vi "duty cycle.vi"(4 "State":i16, 5 "Time":dbl format="%.2f", 6 "Sensor Values":dbl[](array[numeric]), 7 "Set Points":dbl[](array[numeric])) -> (0 "required data":T1={"Set Point names"=["on time (s)", "off time (s)", "on value"], "required number of setpoints"=3, "required number of sensors"=1, "Sensor names"=["elapsed time"]}, 3 "output value":dbl)   [LabVIEW 2010]
panel:
  # "Enter the correct information for this control code in the required data structure below. Then make the current value default by right clicking on the border of the data structure. Select \"data operations\" and then select \"make current value default\". These values will be displayed by process controller."
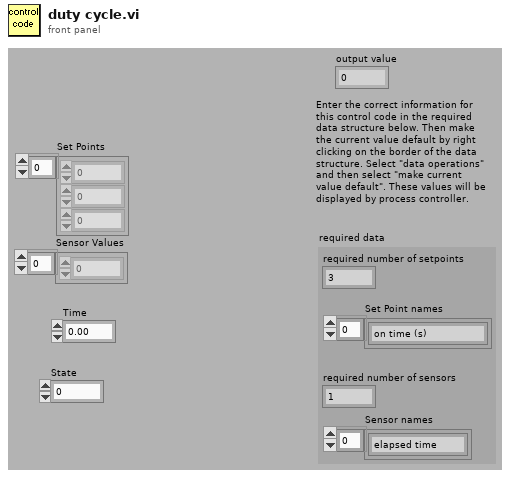
[diagram p1: front panel]
types:
  T1 = cluster{"Set Point names":string[], "required number of setpoints":u8, "required number of sensors":u8, "Sensor names":string[]}
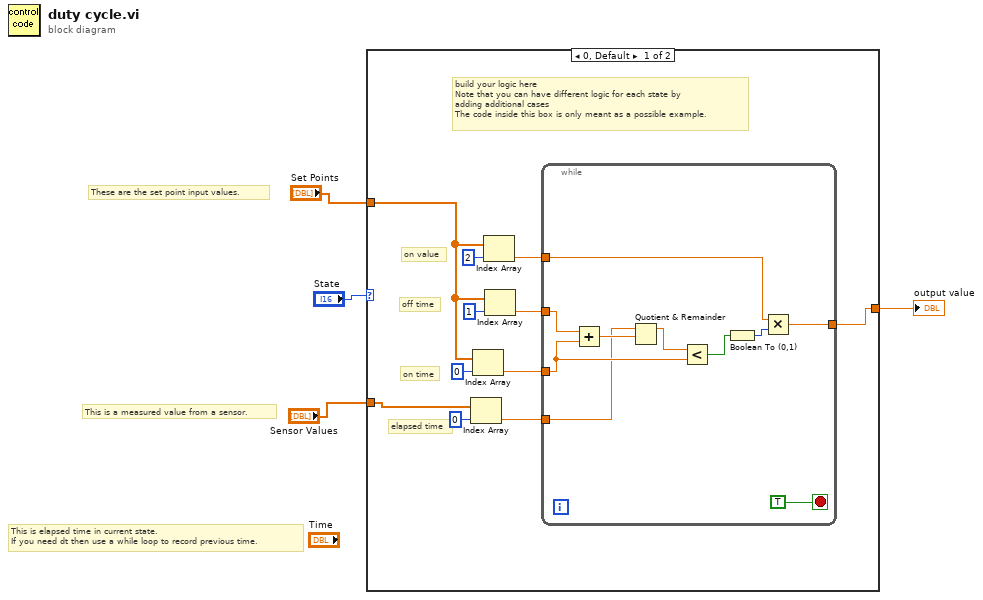
[diagram p0: block diagram]
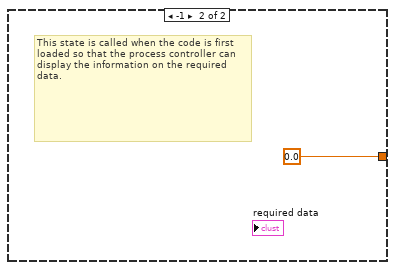
[diagram p2: hidden frame]
diagram:
  # "These are the set point input values."
  # "This is a measured value from a sensor."
  # "This is elapsed time in current state.\nIf you need dt then use a while loop to record previous time."
  n1 = case shown="0, Default" "State" {
    tunnel: [w8 0.0 ("fraction on")] -> w3
    tunnel: "Set Points" -> [w10 _]
    tunnel: "Sensor Values" -> [w6 _]
    frame 0, Default {
      # "elapsed time"
      # "on value"
      # "off time"
      # "on time"
      # "build your logic here\nNote that you can have different logic for each state by\nadding additional cases\nThe code inside this box is only meant as a possible example."
      n2 = Index Array(array=w6, index=0) -> (element=w5:dbl)
      n3 = Index Array(array=w10, index=0) -> (element=w12:dbl)
      n4 = Index Array(array=w10, index=2) -> (element=w9:dbl)
      n5 = Index Array(array=w10, index=1) -> (element=w14:dbl)
      n6 = while {
        tunnel: w14 -> [w24]
        tunnel: w12 -> [w22]
        tunnel: w9 -> [w19]
        tunnel: [w18] -> w8
        tunnel: w5 -> [w16]
        stop <- TRUE stop-if-true
        n7 = Add(x=w24, y=w22) -> (x+y=w23:dbl)
        n8 = Quotient & Remainder(x=w16, y=w23) -> (x-y*floor(x/y)=w21:dbl)  [unwired: 1 out]
        n9 = Less?(x=w21, y=w22) -> (x < y?=w17:bool)
        n10 = Boolean To (0,1)(Boolean=w17) -> (0, 1=w20:i16)
        n11 = Multiply(x=w19, y=w20) -> (x*y=w18:dbl)
      }
    }
    frame -1 {
      # "This state is called when the code is first loaded so that the process controller can display the information on the required data."
    }
  }
  "output value" <- w3
